vi "VISA程序.vi"() -> ()   [LabVIEW 2016]
uses:
  VISA/VISA.lvclass
panel:
  out "消息":string
  in  "通讯配置":T1={"波特率"=9600, "数据比特"=8, "parity (0:none)"=0, "超时"=10000} {"parity (0:none)" items=["None", "Odd", "Even", "Mark", "Space"]}
  in  "VISA资源名称":refnum<visa-resource-name>
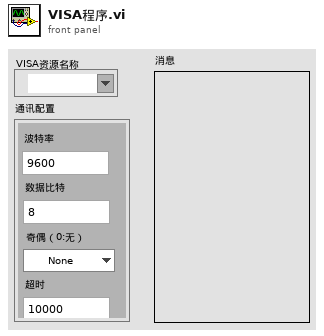
[diagram p1: front panel]
types:
  T1 = cluster{"波特率":u32, "数据比特":u16, "parity (0:none)":u16, "超时":u32}
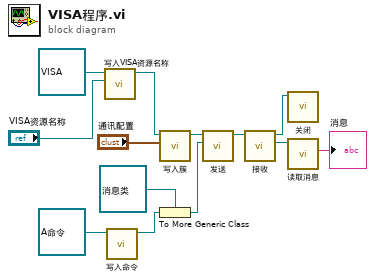
[diagram p0: block diagram]
diagram:
  n1 = call-dynamic "写入VISA资源名称.vi"("VISA资源名称"="VISA资源名称", "VISA输入"=refnum<class "VISA.lvclass"> refnum ("VISA.lvclass")) -> ("VISA输出"=w11:refnum<class "VISA.lvclass">)  [unwired: 8 in, 1 out]
  n2 = call-dynamic "写入命令.vi"("A命令 输入"=refnum<class "A命令.lvclass"> refnum ("A命令.lvclass")) -> ("A命令 输出"=w6:refnum<class "A命令.lvclass">)  [unwired: 9 in, 1 out]
  n3 = call-dynamic "写入簇.vi"("簇"="通讯配置", "VISA输入"=w11) -> ("VISA输出"=w9:refnum<class "VISA.lvclass">)  [unwired: 8 in, 1 out]
  n4 = To More Generic Class(target class=refnum<class "消息类.lvclass"> refnum ("消息类.lvclass"), reference=w6) -> (generic class reference=w4:refnum<class "消息类.lvclass">)
  n5 = call-dynamic "发送.vi"("消息类.lvclass"=w4, "VISA 输入"=w9) -> ("VISA 输出"=w8:refnum<class "VISA.lvclass">)  [unwired: 8 in, 1 out]
  n6 = call-dynamic "接收.vi"("VISA 输入"=w8) -> ("消息类.lvclass"=w2:refnum<class "消息类.lvclass">, "VISA 输出"=w3:refnum<class "VISA.lvclass">)  [unwired: 8 in, 1 out]
  n7 = call-dynamic "关闭.vi"("VISA 输入"=w3) -> ()  [unwired: 10 in, 1 out]
  n8 = call-dynamic "读取消息.vi"("消息类输入"=w2) -> ("消息"=→"消息":string)  [unwired: 8 in, 2 out]
